vi "PS Control.vi"() -> ()   [LabVIEW 2020]
panel:
  in  "Hold":bool
  in  "Ramp to Setpoint":bool
  in  "Slew Rate [T/min]":dbl
  in  "Setpoint [T]":dbl
  in  "Field [T]":dbl step=0.1
  in  "Status":string
  in  "Comments":string
  in  "Æ Trigger":dbl
  in  "Trigger Column":i32
  in  "New/Stop":bool
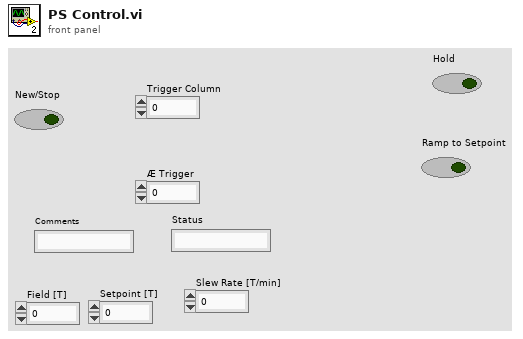
[diagram p1: front panel]
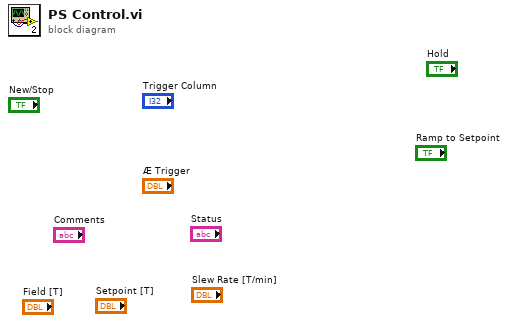
[diagram p0: block diagram]
diagram:
